vi "New.vi"(6 "parent":bool, 7 "icon path":path, 8 "error in (no error)":errorcluster, 11 "item name":string) -> (0 "error out":errorcluster, 3 "text item out":refnum<class "text item.lvclass">)   [LabVIEW 2009, in "text item.lvclass"]
uses:
  text item.lvclass
  text item.lvclass/text item.ctl
  ICON/icon.lvclass
  Text/text.lvclass
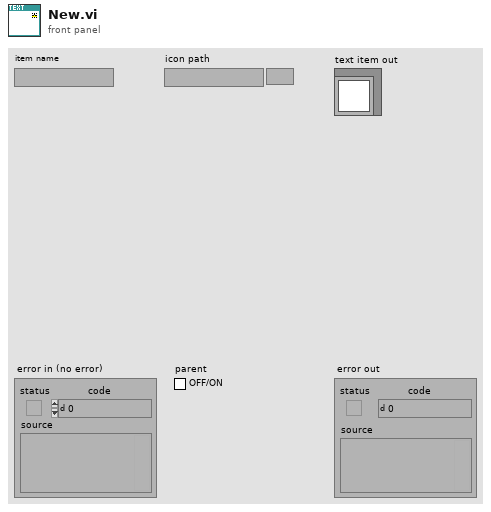
[diagram p1: front panel]
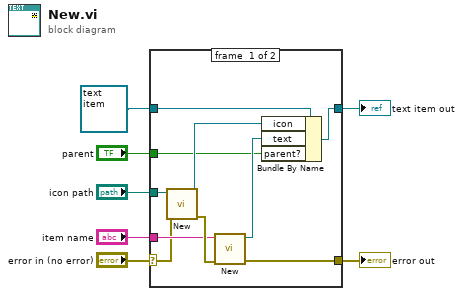
[diagram p0: block diagram]
diagram:
  n1 = case shown="No Error" "error in (no error)" {
    selector: "error in (no error)" -> [w10 w19]
    tunnel: [w9 w19] -> w4
    tunnel: [w16 w18] -> w6
    tunnel: refnum<class "text item.lvclass"> refnum ("text item in") -> [w17 w18]
    tunnel: "item name" -> [w12 _]
    tunnel: "icon path" -> [w11 _]
    tunnel: "parent" -> [w8 _]
    frame #0 {
      n2 = call "New.vi"("error in (no error)"=w10, "icon path"=w11) -> ("error out"=w13:errorcluster, "icon out"=w15:refnum<class "icon.lvclass">)  [unwired: 8 in]
      n3 = call "New.vi"("error in (no error)"=w13, "item name"=w12) -> ("error out"=w9:errorcluster, "text out"=w14:refnum<class "text.lvclass">)  [unwired: 8 in]
      n4 = Bundle By Name(cluster=w17, "icon"=w15, "text"=w14, "parent?"=w8) -> (w16:refnum<class "text item.lvclass">)
    }
    frame #1 {
    }
  }
  "text item out" <- w6
  "error out" <- w4
